vi "CC Script Next Dither.vi"(8 "error in (no error)":errorcluster, 10 "object":T1, 11 "Dither":T6) -> (0 "error out":errorcluster, 1 "Dither?":bool, 2 "object":T1, 3 "Dither out":T6, 4 "Message":string)   [LabVIEW 2021]
uses:
  typedefs/CC cluster Dithering.ctl
  typedefs/CC cluster Random Dithering.ctl
  typedefs/CC Dithering.ctl
  typedefs/CC cluster Offset Dithering.ctl
  typedefs/CC Dithering Offsets.ctl
  typedefs/CC cluster Object.ctl
  typedefs/CC cluster sidereal rate.ctl
  typedefs/CC cluster RA and DEC.ctl
  typedefs/cc cluster muRA muDEC.ctl
  Telescope/CC cluster Telescope Offsets.ctl
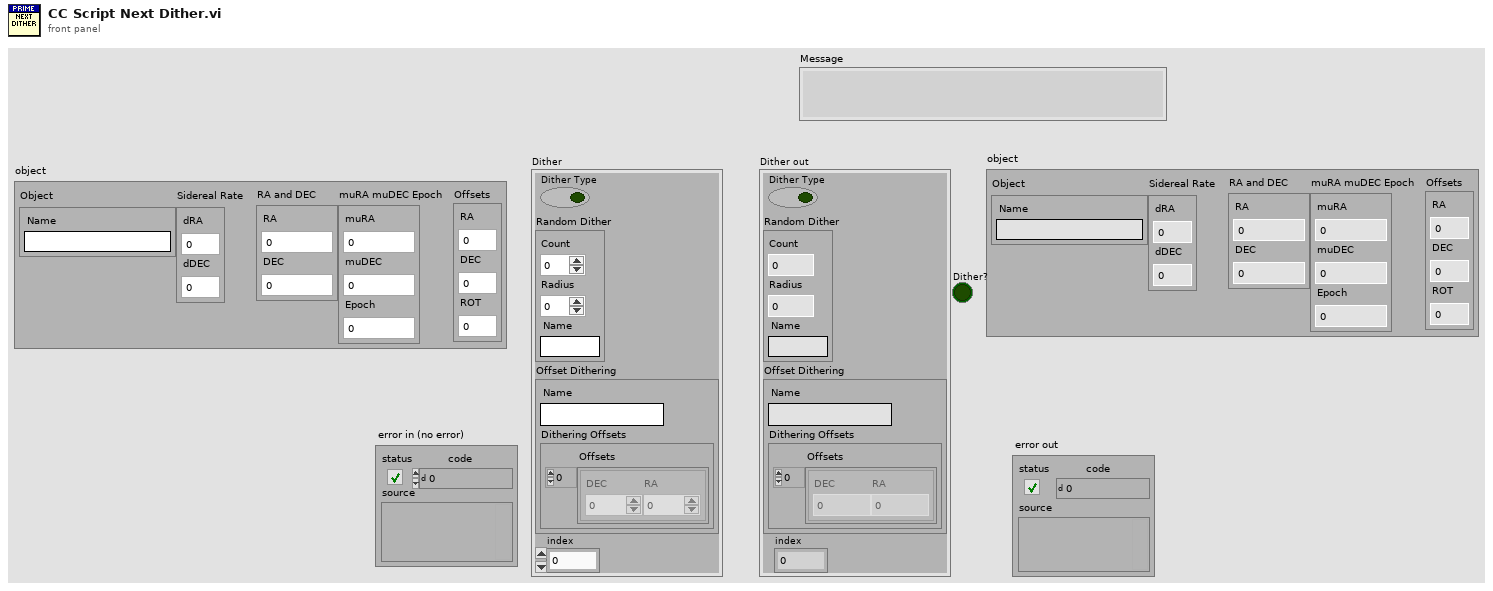
[diagram p1: front panel]
types:
  T1 = typedef "CC cluster Object.ctl" = cluster{"Object":cluster{"Name":string}, "Sidereal Rate":T2, "RA and DEC":T3, "muRA muDEC Epoch":T4, "Offsets":T5}
  T2 = typedef "CC cluster sidereal rate.ctl" = cluster{"dRA":dbl, "dDEC":dbl}
  T3 = typedef "CC cluster RA and DEC.ctl" = cluster{"RA":dbl, "DEC":dbl}
  T4 = typedef "cc cluster muRA muDEC.ctl" = cluster{"muRA":dbl, "muDEC":dbl, "Epoch":dbl}
  T5 = typedef "CC cluster Telescope Offsets.ctl" = cluster{"RA":dbl, "DEC":dbl, "ROT":dbl}
  T6 = typedef "CC cluster Dithering.ctl" = cluster{"Dither Type":bool, "Random Dither":T7, "Offset Dithering":T8, "index":i32}
  T7 = typedef "CC cluster Random Dithering.ctl" = cluster{"Count":i32, "Radius":dbl, "Name":string}
  T8 = typedef "CC Dithering.ctl" = cluster{"Name":string, "Dithering Offsets":T9}
  T9 = typedef "CC cluster Offset Dithering.ctl" = cluster{"Offsets":T10[]}
  T10 = typedef "CC Dithering Offsets.ctl" = cluster{"DEC":dbl, "RA":dbl}
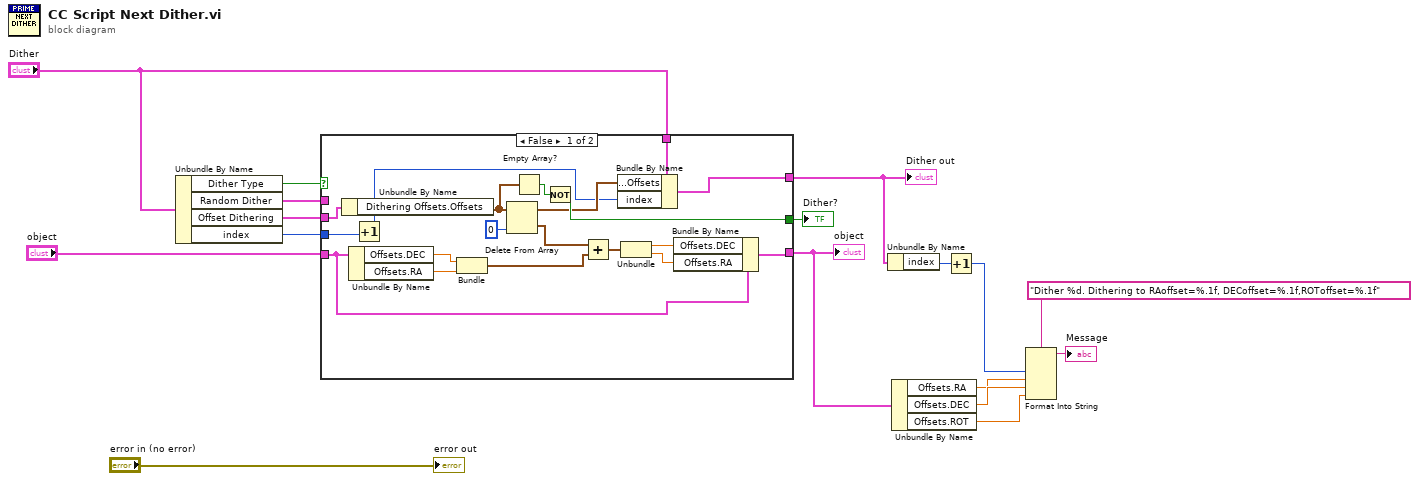
[diagram p0: block diagram]
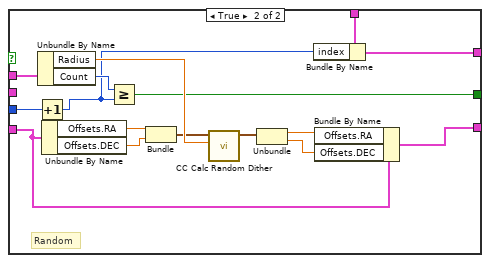
[diagram p2: hidden frame]
diagram:
  n1 = Unbundle By Name("Dither") -> ("Dither Type"=w16:bool, "Random Dither"=w15:T7, "Offset Dithering"=w13:T8, "index"=w14:i32)
  n2 = case shown="False" w16 {
    tunnel: w15 -> [_ w52]
    tunnel: w14 -> [w28 w51]
    tunnel: w13 -> [w36 _]
    tunnel: "object" -> [w22 w40]
    tunnel: [w32 w48] -> w10
    tunnel: [w18 w37] -> w8
    tunnel: "Dither" -> [w31 w46]
    tunnel: [w29 w45] -> w4
    frame False {
      n3 = Unbundle By Name(w36) -> ("Dithering Offsets.Offsets"=w34:T10[])
      n4 = Unbundle By Name(w22) -> ("Offsets.DEC"=w25:dbl, "Offsets.RA"=w26:dbl)
      n5 = Increment(x=w28) -> (x+1=w27:i32)
      n6 = Bundle("DEC"=w25, "RA"=w26) -> (w24:cluster{"DEC":dbl, "RA":dbl})  [unwired: 1 in]
      n7 = Delete From Array(array=w34, index=0) -> (deleted portion=w23:T10, array with subset deleted=w30:T10[])  [unwired: 1 in]
      n8 = Empty Array?(array=w34) -> (empty?=w33:bool)
      n9 = Not(x=w33) -> (.not. x?=w32:bool)
      n10 = Add(x=w23, y=w24) -> (x+y=w21:T10)
      n11 = Bundle By Name(cluster=w31, "Offset Dithering.Dithering Offsets.Offsets"=w30, "index"=w27) -> (w29:T6)
      n12 = Unbundle(w21) -> ("DEC"=w20:dbl, "RA"=w19:dbl)
      n13 = Bundle By Name(cluster=w22, "Offsets.DEC"=w20, "Offsets.RA"=w19) -> (w18:T1)
    }
    frame True {
      # "Random"
      n14 = Increment(x=w51) -> (x+1=w47:i32)
      n15 = Unbundle By Name(w52) -> ("Radius"=w49:dbl, "Count"=w50:i32)
      n16 = Unbundle By Name(w40) -> ("Offsets.RA"=w44:dbl, "Offsets.DEC"=w43:dbl)
      n17 = Greater Or Equal?(x=w50, y=w47) -> (x >= y?=w48:bool)
      n18 = Bundle("RA"=w44, "DEC"=w43) -> (w42:cluster{"RA":dbl, "DEC":dbl})  [unwired: 1 in]
      n19 = call "CC Calc Random Dither.vi"("Radius (arcsec)"=w49, "RA and DEC"=w42) -> ("Dither RA and DEC"=w41:T3)  [unwired: 8 in, 1 out]
      n20 = Unbundle(w41) -> ("RA"=w39:dbl, "DEC"=w38:dbl)
      n21 = Bundle By Name(cluster=w46, "index"=w47) -> (w45:T6)
      n22 = Bundle By Name(cluster=w40, "Offsets.RA"=w39, "Offsets.DEC"=w38) -> (w37:T1)
    }
  }
  "Dither out" <- w4
  "object" <- w8
  "Dither?" <- w10
  n23 = Unbundle By Name(w4) -> ("index"=w2:i32)
  n24 = Unbundle By Name(w8) -> ("Offsets.RA"=w3:dbl, "Offsets.DEC"=w7:dbl, "Offsets.ROT"=w6:dbl)
  n25 = Increment(x=w2) -> (x+1=w1:i32)
  n26 = Format Into String(format string="Dither %d. Dithering to RAoffset=%.1f, DECoffset=%.1f,ROToffset=%.1f", w1, w3, w7, w6) -> (resulting string=→"Message":string)  [unwired: 2 in, 1 out]
  "error out" <- "error in (no error)"
